vi "PXI DAQ TCP Server.vi"(11 "Show stop":bool=TRUE) -> ()   [LabVIEW 2020]
uses:
  DAQ Engine VIs/PXI Globals.vi
panel:
  out "Error":bool
  out "TCP error":errorcluster
  out "data string":string
  out "DAQ in progress":bool
  out "Status":bool
  out "Ready":bool
  out "Busy":bool
  out "Primary":bool
  in  "stop":bool
  out "error out":errorcluster
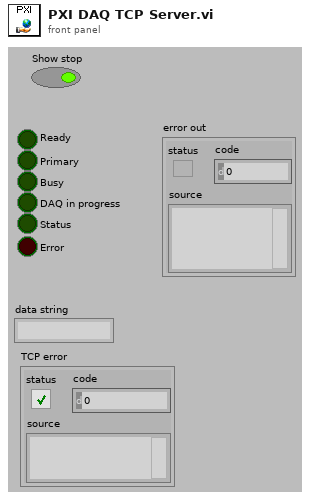
[diagram p1: front panel]
types:
  T1 = cluster{"Major":i32, "Minor":i32, "Build":i32, "Private":i32, "FileVersion":string, "ProductName":string, "InternalName":string, "CompanyName":string, "LegalCopyright":string, "FileDescription":string}
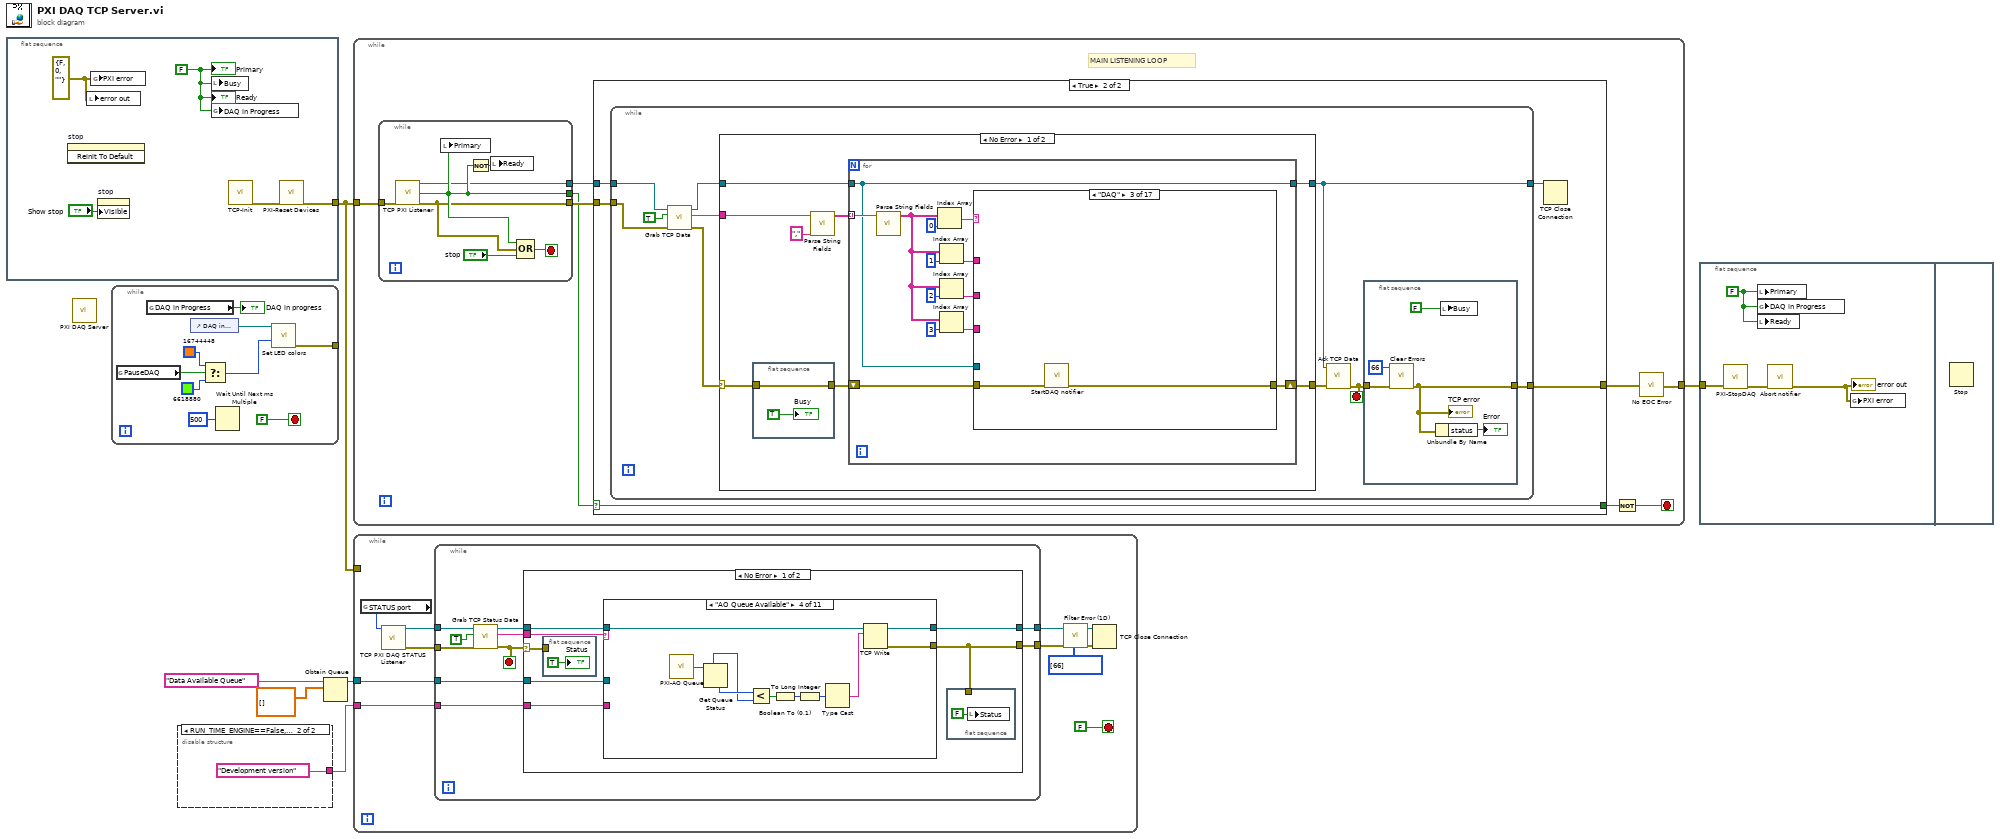
[diagram p0: block diagram]
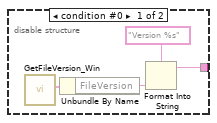
[diagram p2: hidden frame]
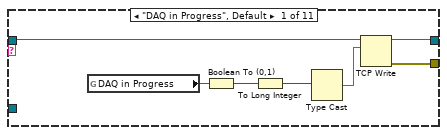
[diagram p3: hidden frame]
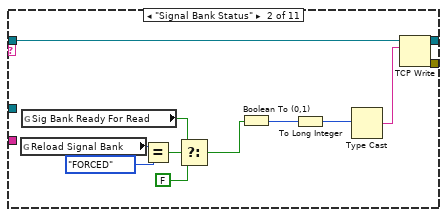
[diagram p4: hidden frame]
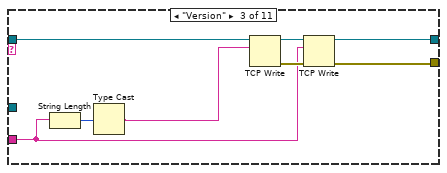
[diagram p5: hidden frame]
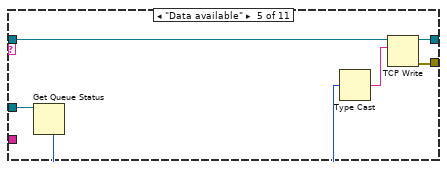
[diagram p6: hidden frame]
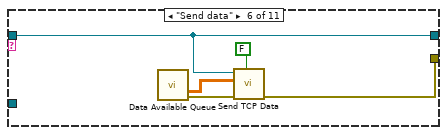
[diagram p7: hidden frame]
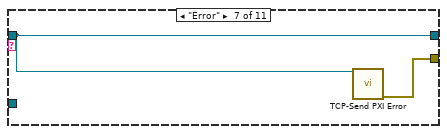
[diagram p8: hidden frame]
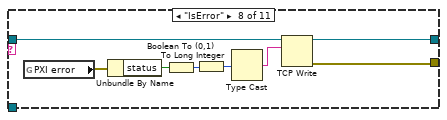
[diagram p9: hidden frame]
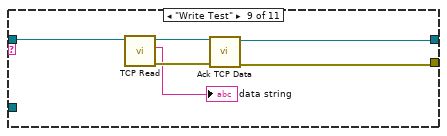
[diagram p10: hidden frame]
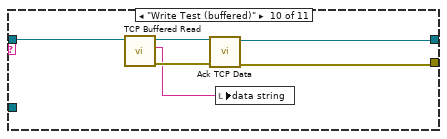
[diagram p11: hidden frame]
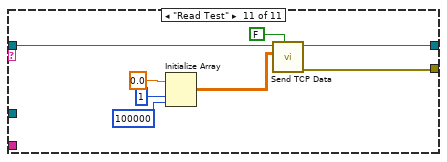
[diagram p12: hidden frame]
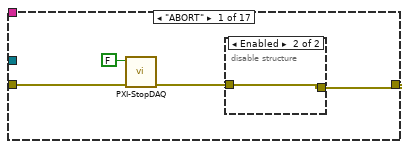
[diagram p15: hidden frame]
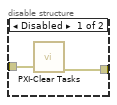
[diagram p16: hidden frame]
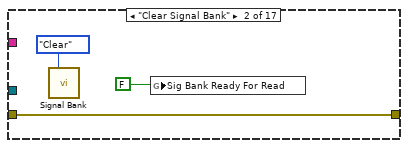
[diagram p17: hidden frame]
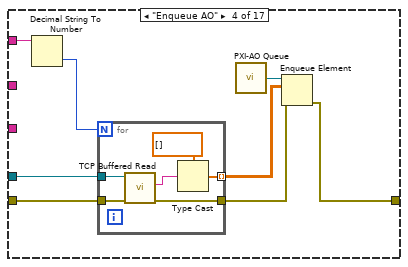
[diagram p18: hidden frame]
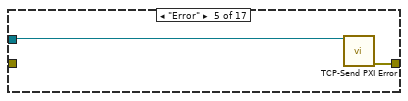
[diagram p19: hidden frame]
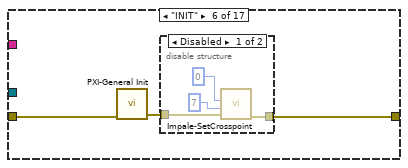
[diagram p20: hidden frame]
diagram:
  n1 = flat-sequence {
    tunnel: [w11] -> w2
    frame #0 {
      w10 = errorcluster {"status"=FALSE, "code"=0, "source"=""} ("PXI error")
      w8 = FALSE ("Connected?")
      n2 = invoke on="stop" class="Bool" method="Reinit To Default"() -> ()  [unwired: 3 in, 3 out]
      n3 = local write "error out"(w10) -> ()
      n4 = global write "PXI Globals.vi" "PXI error"(w10) -> ()
      n5 = property on="stop" class="Bool"("Visible"="Show stop") -> ()  [unwired: 2 in, 2 out]
      n6 = local write "Busy"(w8) -> ()
      n7 = global write "PXI Globals.vi" "DAQ in Progress"(w8) -> ()
      n8 = call "TCP-Init.vi"() -> ("error out"=w9:errorcluster)  [unwired: 15 in]
      n9 = call "PXI-Reset Devices.vi"("error in"=w9) -> ("error out"=w11:errorcluster)  [unwired: 10 in]
      "Primary" <- w8
      "Ready" <- w8
    }
  }
  n10 = call "PXI DAQ Server.vi"() -> ()  [unwired: 7 in, 1 out]
  n11 = while {
    tunnel: [w13] -> _
    stop <- FALSE stop-if-true
    n12 = global read "PXI Globals.vi" "PauseDAQ"() -> (w16:bool)
    n13 = global read "PXI Globals.vi" "DAQ in Progress"() -> (→"DAQ in progress":bool)
    n14 = control-ref of="DAQ in progress"() -> (w17:refnum<vi>)
    n15 = Select(t=u32 16744448, s=w16, f=u32 6618880) -> (s? t:f=w12:u32)
    n16 = Wait Until Next ms Multiple(millisecond multiple=500) -> ()  [unwired: 1 out]
    n17 = call "Set LED colors.vi"("On color"=w12, "reference"=w17) -> ("error out"=w13:errorcluster)  [unwired: 8 in, 1 out]
  }
  n18 = disable-structure shown="RUN_TIME_ENGINE==False, Default" {
    disable-tunnel: [w22 "Development version" ("format string")] -> w1
    frame condition #0 {
      n19 = call "GetFileVersion_Win.vi"() -> ("File Info Out"=w23:T1)  [unwired: 9 in, 2 out]
      n20 = Unbundle By Name(w23) -> ("FileVersion"=w21:string)
      n21 = Format Into String(format string="Version %s", w21) -> (resulting string=w22:string)  [unwired: 2 in, 1 out]
    }
    frame condition #1 (active) {
    }
  }
  n22 = Obtain Queue(name (unnamed)="Data Available Queue", element data type=dbl[][] [] ("AI Waveforms 2")) -> (queue out=w3:refnum<queue>)  [unwired: 3 in, 2 out]
  n23 = while {
    tunnel: [w28] -> w6
    tunnel: w2 -> [w31]
    stop <- w27 stop-if-true
    # "MAIN LISTENING LOOP"
    n24 = while {
      tunnel: [w214] -> w33
      tunnel: w31 -> [w220]
      tunnel: [w216] -> w30
      tunnel: [w215] -> w26
      stop <- w218 stop-if-true
      n25 = call "TCP PXI Listener.vi"("error in (no error)"=w220) -> ("connection ID"=w215:refnum<k5>, "Connected?"=w216:bool, "error out"=w214:errorcluster)  [unwired: 12 in]
      n26 = local write "Primary"(w216) -> ()
      n27 = Not(x=w216) -> (.not. x?=w217:bool)
      n28 = local write "Ready"(w217) -> ()
      n29 = Compound Arithmetic op=OR(w216, w214, "stop") -> (w218:bool)
    }
    n30 = case shown="True" w30 {
      selector: w30 -> [w34 w39]
      tunnel: [w35 w38] -> w32
      tunnel: w33 -> [w35 w40]
      tunnel: [w34 w39] -> w29
      tunnel: w26 -> [_ w37]
      frame False {
      }
      frame True {
        n31 = while {
          tunnel: w40 -> [w50]
          tunnel: [w47] -> w38
          tunnel: w37 -> [w44]
          tunnel: [w42] -> w36
          stop <- w41 stop-if-true
          n32 = call "Grab TCP Data.vi"("connection ID"=w44, "No timeout?"=TRUE, "error in (no error)"=w50) -> ("connection ID 2"=w43:refnum<k5>, "data out"=w49:string, "error out"=w46:errorcluster)  [unwired: 5 in]
          n33 = case shown="No Error" w46 {
            selector: w46 -> [w58 w213]
            tunnel: [w60 w213] -> w48
            tunnel: w49 -> [w63 _]
            tunnel: w43 -> [w57 w212]
            tunnel: [w56 w212] -> w42
            frame No Error {
              n34 = flat-sequence {
                tunnel: w58 -> [w64]
                tunnel: [w64] -> w59
                frame #0 {
                  "Busy" <- TRUE ("Receiving")
                }
              }
              n35 = call "Parse String Fields.vi"("Separator"=",", "String"=w63) -> ("Fields"=w61:string[])  [unwired: 8 in, 1 out]
              n36 = for {
                tunnel: w61 -> [w67] mode=indexing
                shift-right: [w77] -> w60
                shift-left: w59 -> [w78]
                tunnel: w57 -> [w66]
                tunnel: [w66] -> w56
                n37 = call "Parse String Fields.vi"("String"=w67) -> ("Fields"=w68:string[])  [unwired: 9 in, 1 out]
                n38 = Index Array(array=w68, index=0) -> (element=w75:string)
                n39 = Index Array(array=w68, index=1) -> (element=w71:string)
                n40 = Index Array(array=w68, index=2) -> (element=w72:string)
                n41 = Index Array(array=w68, index=3) -> (element=w69:string)
                n42 = case shown="\"DAQ\"" w75 {
                  selector: w75 -> [_ _ _ _ _ _ _ _ _ _ _ _ _ _ _ _ w204]
                  tunnel: w78 -> [w81 w88 w89 w95 _ w107 w115 w119 w123 w129 w149 w159 w164 w167 w189 w202 w210]
                  tunnel: [w82 w88 w90 w97 w106 w109 w115 w119 w122 w130 w146 w159 w161 w169 w188 w202 w203] -> w77
                  tunnel: w72 -> [_ _ _ _ _ _ _ _ w121 w127 _ _ w163 w166 w187 _ _]
                  tunnel: w71 -> [_ _ _ w92 _ _ _ w117 _ _ _ _ _ w168 _ _ _]
                  tunnel: w69 -> [_ _ _ _ _ _ _ _ w120 w124 w147 _ w162 w165 _ _ _]
                  tunnel: w66 -> [_ _ _ w96 w105 _ _ _ _ w125 w148 _ _ _ _ _ _]
                  frame "ABORT" {
                    n43 = call "PXI-StopDAQ.vi"("error in (no error)"=w81, "Wait for DAQ to stop? (T)"=FALSE) -> ("error out"=w80:errorcluster)  [unwired: 5 in]
                    n44 = disable-structure shown="Enabled" {
                      disable-tunnel: w80 -> [w84 w85]
                      disable-tunnel: [w83 w85] -> w82
                      frame Disabled {
                        n45 = call "PXI-Clear Tasks.vi"("error in (no error)"=w84) -> ("error out"=w83:errorcluster)  [unwired: 14 in]
                      }
                      frame Enabled {
                      }
                    }
                  }
                  frame "Clear Signal Bank" {
                    n46 = call "Signal Bank.vi"("Action"=enum16{"Add", "Replace ID", "Read ID", "Clear"}."Clear") -> ()  [unwired: 13 in, 2 out]
                    n47 = global write "PXI Globals.vi" "Sig Bank Ready For Read"(FALSE ("DAQ Connected")) -> ()
                  }
                  frame "DAQ" {
                    n48 = call "StartDAQ notifier.vi"("error in (no error)"=w89) -> ("error out"=w90:errorcluster)  [unwired: 6 in]
                  }
                  frame "Enqueue AO" {
                    n49 = Decimal String To Number(string=w92) -> (number=w91:i32)  [unwired: 2 in, 1 out]
                    n50 = for {
                      N: w91 -> [_]
                      tunnel: w96 -> [w104]
                      tunnel: w95 -> [w103]
                      tunnel: [w100] -> w93 mode=indexing
                      tunnel: [w99] -> w94
                      n51 = call "TCP Buffered Read.vi"("error in (no error)"=w103, "connection ID"=w104) -> ("error out"=w99:errorcluster, "data string"=w101:string)  [unwired: 6 in, 2 out]
                      n52 = Type Cast(type=dbl[] [], x=w101) -> (*(type *) &x=w100:dbl[])
                    }
                    n53 = call "PXI-AO Queue.vi"() -> ("Queue"=w98:refnum<queue>)  [unwired: 15 in]
                    n54 = Enqueue Element(queue=w98, element=w93, error in (no error)=w94) -> (error out=w97:errorcluster)  [unwired: 1 in, 2 out]
                  }
                  frame "Error" {
                    n55 = call "TCP-Send PXI Error.vi"("connection ID"=w105) -> ("error out"=w106:errorcluster)  [unwired: 14 in]
                  }
                  frame "INIT" {
                    n56 = call "PXI-General Init.vi"("error in (no error)"=w107) -> ("error out"=w108:errorcluster)  [unwired: 10 in]
                    n57 = disable-structure shown="Disabled" {
                      disable-tunnel: [w113 w114] -> w109
                      disable-tunnel: w108 -> [w110 w114]
                      frame Disabled {
                        n58 = call "Impale-SetCrosspoint.vi"("error in (no error)"=w110, "Site"=7, "Bank"=0) -> ("error out"=w113:errorcluster)  [unwired: 4 in]
                      }
                      frame Enabled {
                      }
                    }
                  }
                  frame "NOOP" {
                    # "// do nothing"
                  }
                  frame "Pause" {
                    n59 = Decimal String To Number(string=w117) -> (number=w118:i32)  [unwired: 2 in, 1 out]
                    n60 = Not Equal To 0?(x=w118) -> (x != 0?=w116:bool)
                    n61 = global write "PXI Globals.vi" "PauseDAQ"(w116) -> ()
                  }
                  frame "SETKEY" {
                    n62 = call "TCP-Parse Key.vi"("error in (no error)"=w123, "Value"=w120, "Key"=w121) -> ("error out"=w122:errorcluster)  [unwired: 8 in]
                  }
                  frame "SETWAVE" {
                    n63 = case shown="\"BUF\"" w124 {
                      tunnel: w129 -> [w134 w138]
                      tunnel: [w133 w137] -> w128
                      tunnel: [w132 w136] -> w126
                      tunnel: w125 -> [w131 w135]
                      frame "BUF" {
                        n64 = call "TCP Buffered Read.vi"("error in (no error)"=w134, "connection ID"=w131) -> ("error out"=w132:errorcluster, "data string"=w133:string)  [unwired: 6 in, 2 out]
                      }
                      frame "UNBUF", Default {
                        n65 = call "TCP Read.vi"("error in (no error)"=w138, "connection ID"=w135) -> ("error out"=w136:errorcluster, "data string"=w137:string)  [unwired: 7 in, 1 out]
                      }
                    }
                    n66 = case shown="No Error" w126 {
                      selector: w126 -> [w139 w145]
                      tunnel: [w139 w145] -> w130
                      tunnel: w128 -> [w143 _]
                      tunnel: w127 -> [w140 _]
                      frame No Error {
                        # "all WAVEs are assumed\nto be binary DOUBLEs"
                        n67 = Type Cast(type=dbl[] [], x=w143) -> (*(type *) &x=w141:dbl[])
                        n68 = call "Signal Bank.vi"("Action"=enum16{"Add", "Replace ID", "Read ID", "Clear"}."Add", "1D Data In"=w141, "ID"=w140) -> ()  [unwired: 11 in, 2 out]
                      }
                      frame Error {
                      }
                    }
                  }
                  frame "BufferedWriteTest" {
                    n69 = case shown="\"BUF\"" w147 {
                      tunnel: w149 -> [w154 w158]
                      tunnel: [w153 w157] -> _
                      tunnel: [w152 w156] -> w146
                      tunnel: w148 -> [w151 w155]
                      frame "BUF" {
                        n70 = call "TCP Buffered Read.vi"("error in (no error)"=w154, "timeout (ms)"=1000, "connection ID"=w151) -> ("error out"=w152:errorcluster, "data string"=w153:string)  [unwired: 5 in, 2 out]
                      }
                      frame "UNBUF", Default {
                        n71 = call "TCP Read.vi"("error in (no error)"=w158, "connection ID"=w155) -> ("error out"=w156:errorcluster, "data string"=w157:string)  [unwired: 7 in, 1 out]
                      }
                    }
                  }
                  frame "STOPDAQ" {
                    n72 = global write "PXI Globals.vi" "StopDAQ"(TRUE) -> ()
                  }
                  frame "Set Multipliers" {
                    n73 = call "TCP-Set AO Gains.vi"("error in (no error)"=w164, "Gain String"=w162, "Channel String"=w163) -> ("error out"=w161:errorcluster)  [unwired: 8 in]
                  }
                  frame "SetAOGains" {
                    n74 = case shown="No Error" w167 {
                      selector: w167 -> [w175 w179]
                      tunnel: [w172 w179] -> w169
                      tunnel: w168 -> [w173 _]
                      tunnel: w166 -> [w171 _]
                      tunnel: w165 -> [w170 _]
                      frame No Error {
                        n75 = call "TCP-Set AO Gains.vi"("error in (no error)"=w175, "Gain String"=w170, "Channel String"=w171) -> ("error out"=w174:errorcluster)  [unwired: 8 in]
                        n76 = case shown="\"OTF\"" w173 {
                          tunnel: w174 -> [w176 w178]
                          tunnel: [w176 w177] -> w172
                          frame "False", Default {
                          }
                          frame "OTF" {
                            n77 = call "PXI-Set AO Gains OTF.vi"("error in (no error)"=w178) -> ("error out"=w177:errorcluster)  [unwired: 10 in]
                          }
                        }
                      }
                      frame Error {
                      }
                    }
                  }
                  frame "TRIG" {
                    n78 = Obtain Notifier(name (unnamed)=w187, notification data type=FALSE, error in (no error)=w189) -> (notifier out=w185:refnum<notifier>, error out=w184:errorcluster)  [unwired: 1 in, 1 out]
                    n79 = Get Notifier Status(notifier=w185, error in (no error)=w184) -> (notifier out=w181:refnum<notifier>, # waiting=w183:i32, error out=w180:errorcluster)  [unwired: 2 out]
                    n80 = Greater Than 0?(x=w183) -> (x > 0?=w182:bool)
                    n81 = case shown="True" w182 {
                      tunnel: [w190 w199] -> w188
                      tunnel: w181 -> [w192 w196]
                      tunnel: w180 -> [w191 w195]
                      tunnel: w187 -> [_ w194]
                      frame False {
                        # "// no one is waiting\n// on this trigger,\n// so ignore it"
                        n82 = Release Notifier(notifier=w192, force destroy? (F)=TRUE, error in (no error)=w191) -> (error out=w190:errorcluster)  [unwired: 2 out]
                      }
                      frame True {
                        n83 = case shown="\"StartDAQ\"" w194 {
                          frame Default {
                          }
                          frame "StartDAQ" {
                            # "Set DAQ in Progress here to make sure it's set for next call to  TCP Grab"
                            n84 = global write "PXI Globals.vi" "DAQ in Progress"(TRUE ("DAQ in Progress")) -> ()
                          }
                        }
                        n85 = Unbundle By Name(w195) -> ("status"=w198:bool)
                        n86 = Not(x=w198) -> (.not. x?=w197:bool)
                        n87 = Send Notification(notification=w197, notifier=w196, error in (no error)=w195) -> (error out=w199:errorcluster)  [unwired: 1 out]
                      }
                    }
                  }
                  frame "WAVEREADY" {
                    n88 = global write "PXI Globals.vi" "Sig Bank Ready For Read"(TRUE) -> ()
                  }
                  frame Default {
                    w209 = 1 items=["No error", "Argument error", "Memory is full", "Out of zone", "End of file", "File already open", "Generic file I/O error", "File not found", "File permission error", "Disk is full", "Duplicate path", "Too many files open", "System feature not enabled", "Resource file not found", "Cannot add resource", "Resource not found", "Image not found", "Image memory error", "Pen does not exist", "Config type invalid", "Config token not found", "Config parse error", "Config memory error", "Bad external code format", "Bad external code offset", "External code not present", "Null window", "Destroy window error", "Null menu", "Print aborted", "Bad print record", "Print driver error", "Windows error during printing", "Memory error during printing", "Print dialog error", "Generic print error", "Invalid device refnum", "Device not found", "Device parameter error", "Device unit error", "Cannot open device", "Device call aborted", "Generic error", "Cancelled by user", "Object ID too low", "Object ID too high", "Object not in heap", "Unknown heap", "Unknown object (invalid DefProc)", "Unknown object (DefProc not in table)", "Message out of range", "Invalid (null) method", "Unknown message", "Manager call not supported", "Bad address", "Network operation in progress", "Network operation timed out", "Connection is busy", "Network attribute not supported", "Network error", "Address in use", "System out of memory", "Connection aborted", "Connection refused", "Not connected", "Already connected", "Connection closed", "Initialization error (interapplication manager)", "Bad occurrence", "Wait on unbound occurrence handler", "Occurrence queue overflow", "Datalog type conflict", "Unused", "Unrecognized type (interapplication manager)", "Memory corrupt", "Failed to make temporary DLL", "Old CIN version", "Drag socket not found", "Failed to load drop-object", "Failed to register OLE object", "Failed to release OLE object", "Format specifier type mismatch", "Unknown format specifier", "Too few format specifiers", "Too many format specifiers", "Scan failed", "Newer CIN version", "Error converting to variant", "Runtime menu error", "Password tampered", "Variant attribute not found", "Incompatible variant data type", "Event data is not available", "Event Store is not present", "Occurrence is not found", "Event Queue is not created", "Event info is not available", "Refnum passed is NULL", "Error retrieving Class GUID", "Error retrieving CoClass GUID", "Error retrieving TypeLib GUID.", "Bad built application magic bytes.", "Specific driver is different from the specific driver associated with the Logical Name.", "There is no session opened to the class driver.", "Max Error", "MAX - Error with config objects", "MAX - Error loading configuration", "MAX - Group not supported"]
                    n89 = Current VI's Path() -> (path=w207:path)
                    n90 = Strip Path(path=w207) -> (name=w206:string)  [unwired: 1 out]
                    n91 = Format Into String(format string="%s: unrecognized TCP tag '%s'", w206, w204) -> (resulting string=w211:string)  [unwired: 2 in, 1 out]
                    n92 = Bundle By Name(cluster=w210, "code"=w209, "status"=TRUE, "source"=w211) -> (w203:errorcluster)
                  }
                }
              }
            }
            frame Error {
            }
          }
          n93 = call "Ack TCP Data.vi"("connection ID"=w42, "error in (no error)"=w48) -> ("error out"=w41:errorcluster)  [unwired: 7 in, 1 out]
          n94 = flat-sequence {
            tunnel: w41 -> [w53]
            tunnel: [w52] -> w47
            frame #0 {
              n95 = call <vilib>:"Clear Errors.vi"("error in (no error)"=w53, "specific error code to clear (0: all)"=66) -> ("error out"=w52:errorcluster)  [unwired: 4 in, 1 out]
              "TCP error" <- w52
              n96 = Unbundle By Name(w52) -> ("status"=→"Error":bool)
              n97 = local write "Busy"(FALSE ("Receiving")) -> ()
            }
          }
        }
        n98 = TCP Close Connection(connection ID=w36) -> ()  [unwired: 2 in, 2 out]
      }
    }
    n99 = Not(x=w29) -> (.not. x?=w27:bool)
    n100 = call "No EOC Error.vi"("error in"=w32) -> ("error out"=w28:errorcluster)  [unwired: 4 in]
  }
  n101 = while {
    tunnel: w3 -> [w227]
    tunnel: w2 -> [_]
    tunnel: w1 -> [w221]
    stop <- FALSE stop-if-true
    n102 = global read "PXI Globals.vi" "STATUS port"() -> (w228:u16)
    n103 = call "TCP PXI DAQ STATUS Listener.vi"("port"=w228) -> ("connection ID"=w226:refnum<k5>, "error out"=w230:errorcluster)  [unwired: 12 in, 1 out]
    n104 = while {
      tunnel: w230 -> [w239]
      tunnel: [w238] -> w225
      tunnel: w227 -> [w237]
      tunnel: w226 -> [w235]
      tunnel: [w232] -> w224
      tunnel: w221 -> [w231]
      stop <- w233 stop-if-true
      n105 = call "Grab TCP Status Data.vi"("connection ID"=w235, "No timeout?"=TRUE, "error in (no error)"=w239) -> ("Status ID out"=w234:refnum<k5>, "data out"=w240:string, "error out"=w233:errorcluster)  [unwired: 5 in]
      n106 = case shown="No Error" w233 {
        selector: w233 -> [w242 w329]
        tunnel: w240 -> [w247 _]
        tunnel: [w243 w329] -> w238
        tunnel: w237 -> [w246 _]
        tunnel: w234 -> [w245 w328]
        tunnel: [w244 w328] -> w232
        tunnel: w231 -> [w241 _]
        frame No Error {
          n107 = flat-sequence {
            tunnel: w242 -> [_]
            frame #0 {
              "Status" <- TRUE ("Status")
            }
          }
          n108 = case shown="\"AO Queue Available\"" w247 {
            tunnel: [w253 w265 w271 w285 w291 w294 w299 w302 w310 w319 w320] -> w243
            tunnel: w246 -> [_ _ _ _ w290 _ _ _ _ _ _]
            tunnel: w245 -> [w251 w258 w275 w284 w288 w293 w298 w301 w313 w317 w327]
            tunnel: [w250 w257 w273 w283 w287 w293 w298 w300 w309 w318 w326] -> w244
            tunnel: w241 -> [_ _ w269 _ _ _ _ _ _ _ _]
            frame "DAQ in Progress", Default {
              n109 = global read "PXI Globals.vi" "DAQ in Progress"() -> (w252:bool)
              n110 = Boolean To (0,1)(Boolean=w252) -> (0, 1=w255:i16)
              n111 = To Long Integer(number=w255) -> (32bit integer=w254:i32)
              n112 = Type Cast(x=w254) -> (*(type *) &x=w256:string)  [unwired: 1 in]
              n113 = TCP Write(connection ID=w251, data in=w256) -> (connection ID out=w250:refnum<k5>, error out=w253:errorcluster)  [unwired: 2 in, 1 out]
            }
            frame "Signal Bank Status" {
              n114 = global read "PXI Globals.vi" "Reload Signal Bank"() -> (w264:enum32{"OFF", "ENABLED", "FORCED"})
              n115 = global read "PXI Globals.vi" "Sig Bank Ready For Read"() -> (w261:bool)
              n116 = Equal?(x=w264, y=enum32{"OFF", "ENABLED", "FORCED"}."FORCED") -> (x = y?=w262:bool)
              n117 = Select(t=w261, s=w262, f=FALSE) -> (s? t:f=w259:bool)
              n118 = Boolean To (0,1)(Boolean=w259) -> (0, 1=w267:i16)
              n119 = To Long Integer(number=w267) -> (32bit integer=w266:i32)
              n120 = Type Cast(x=w266) -> (*(type *) &x=w268:string)  [unwired: 1 in]
              n121 = TCP Write(connection ID=w258, data in=w268) -> (connection ID out=w257:refnum<k5>, error out=w265:errorcluster)  [unwired: 2 in, 1 out]
            }
            frame "Version" {
              n122 = String Length(string=w269) -> (length=w276:i32)
              n123 = Type Cast(x=w276) -> (*(type *) &x=w270:string)  [unwired: 1 in]
              n124 = TCP Write(connection ID=w275, data in=w270) -> (connection ID out=w274:refnum<k5>, error out=w272:errorcluster)  [unwired: 2 in, 1 out]
              n125 = TCP Write(connection ID=w274, data in=w269, error in (no error)=w272) -> (connection ID out=w273:refnum<k5>, error out=w271:errorcluster)  [unwired: 1 in, 1 out]
            }
            frame "AO Queue Available" {
              n126 = call "PXI-AO Queue.vi"() -> ("Queue"=w282:refnum<queue>)  [unwired: 15 in]
              n127 = Get Queue Status(queue=w282) -> (max queue size=w280:i32, # elements in queue=w281:i32)  [unwired: 2 in, 6 out]
              n128 = Less?(x=w281, y=w280) -> (x < y?=w279:bool)
              n129 = Boolean To (0,1)(Boolean=w279) -> (0, 1=w278:i16)
              n130 = To Long Integer(number=w278) -> (32bit integer=w277:i32)
              n131 = Type Cast(x=w277) -> (*(type *) &x=w286:string)  [unwired: 1 in]
              n132 = TCP Write(connection ID=w284, data in=w286) -> (connection ID out=w283:refnum<k5>, error out=w285:errorcluster)  [unwired: 2 in, 1 out]
            }
            frame "Data available" {
              n133 = Get Queue Status(queue=w290) -> (# elements in queue=w289:i32)  [unwired: 2 in, 7 out]
              n134 = Type Cast(x=w289) -> (*(type *) &x=w292:string)  [unwired: 1 in]
              n135 = TCP Write(connection ID=w288, data in=w292) -> (connection ID out=w287:refnum<k5>, error out=w291:errorcluster)  [unwired: 2 in, 1 out]
            }
            frame "Send data" {
              n136 = call "Data Available Queue.vi"() -> ("AI Waveforms"=w296:dbl[][], "error out"=w295:errorcluster)  [unwired: 11 in, 3 out]
              n137 = call "Send TCP Data.vi"("connection ID"=w293, "Data in"=w296, "error in (no error)"=w295, "Single precision?"=FALSE) -> ("error out"=w294:errorcluster)  [unwired: 5 in, 1 out]
            }
            frame "Error" {
              n138 = call "TCP-Send PXI Error.vi"("connection ID"=w298) -> ("error out"=w299:errorcluster)  [unwired: 14 in]
            }
            frame "IsError" {
              n139 = global read "PXI Globals.vi" "PXI error"() -> (w306:errorcluster)
              n140 = Unbundle By Name(w306) -> ("status"=w305:bool)
              n141 = Boolean To (0,1)(Boolean=w305) -> (0, 1=w304:i16)
              n142 = To Long Integer(number=w304) -> (32bit integer=w303:i32)
              n143 = Type Cast(x=w303) -> (*(type *) &x=w307:string)  [unwired: 1 in]
              n144 = TCP Write(connection ID=w301, data in=w307) -> (connection ID out=w300:refnum<k5>, error out=w302:errorcluster)  [unwired: 2 in, 1 out]
            }
            frame "Write Test" {
              n145 = call "TCP Read.vi"("connection ID"=w313) -> ("error out"=w311:errorcluster, "data string"=→"data string":string, "connection ID 2"=w312:refnum<k5>)  [unwired: 8 in]
              n146 = call "Ack TCP Data.vi"("connection ID"=w312, "error in (no error)"=w311) -> ("connection ID out"=w309:refnum<k5>, "error out"=w310:errorcluster)  [unwired: 7 in]
            }
            frame "Write Test (buffered)" {
              n147 = call "TCP Buffered Read.vi"("connection ID"=w317) -> ("error out"=w315:errorcluster, "data string"=w314:string, "connection ID 2"=w316:refnum<k5>)  [unwired: 7 in, 1 out]
              n148 = call "Ack TCP Data.vi"("connection ID"=w316, "error in (no error)"=w315) -> ("connection ID out"=w318:refnum<k5>, "error out"=w319:errorcluster)  [unwired: 7 in]
              n149 = local write "data string"(w314) -> ()
            }
            frame "Read Test" {
              n150 = Initialize Array(0.0 ("element"), 1 ("dimension size"), 100000 ("dimension size")) -> (w321:dbl[][])
              n151 = call "Send TCP Data.vi"("connection ID"=w327, "Data in"=w321, "Single precision?"=FALSE) -> ("connection ID 2"=w326:refnum<k5>, "error out"=w320:errorcluster)  [unwired: 6 in]
            }
          }
          n152 = flat-sequence {
            tunnel: w243 -> [_]
            frame #0 {
              n153 = local write "Status"(FALSE ("Status")) -> ()
            }
          }
        }
        frame Error {
        }
      }
    }
    n154 = call "Filter Error (1D).vi"("error in (no error)"=w225, "Array"=i32[] [66]) -> ("error out"=w223:errorcluster)  [unwired: 9 in]
    n155 = TCP Close Connection(connection ID=w224, error in (no error)=w223) -> ()  [unwired: 1 in, 2 out]
  }
  n156 = flat-sequence {
    tunnel: w6 -> [w332]
    frame #0 {
      w333 = FALSE ("DAQ in Progress")
      n157 = call "PXI-StopDAQ.vi"("error in (no error)"=w332) -> ("error out"=w331:errorcluster)  [unwired: 6 in]
      n158 = local write "Primary"(w333) -> ()
      n159 = global write "PXI Globals.vi" "DAQ in Progress"(w333) -> ()
      n160 = local write "Ready"(w333) -> ()
      n161 = call "Abort notifier.vi"("error in (no error)"=w331) -> ("error out"=w330:errorcluster)  [unwired: 5 in, 1 out]
      "error out" <- w330
      n162 = global write "PXI Globals.vi" "PXI error"(w330) -> ()
    }
    frame #1 {
      n163 = Stop() -> ()  [unwired: 1 in]
    }
  }
